vi "Write PinMap.vi"(8 "error in (no error)":errorcluster, 10 "PinMap":path, 11 "BML_DigiPattern_Generator in":refnum<class "DigiPattern_Generator.lvclass">) -> (0 "error out":errorcluster, 3 "BML_DigiPattern_Generator out":refnum<class "DigiPattern_Generator.lvclass">)   [LabVIEW 2018, in "DigiPattern_Generator.lvclass"]
uses:
  DigiPattern_Generator.lvclass
  DigiPattern_Generator.lvclass/DigiPattern_Generator.ctl
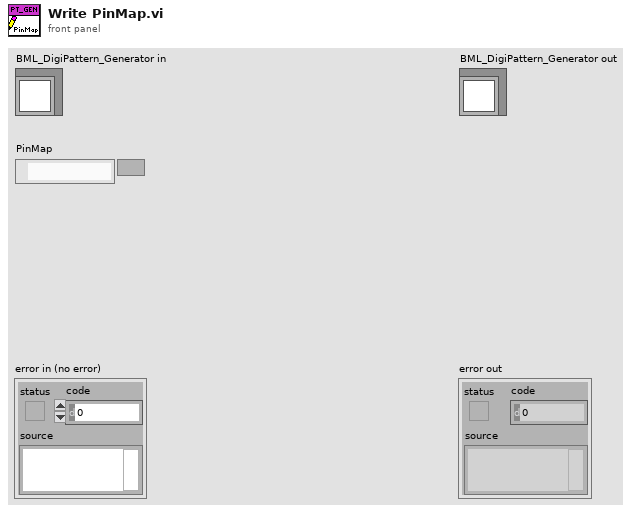
[diagram p1: front panel]
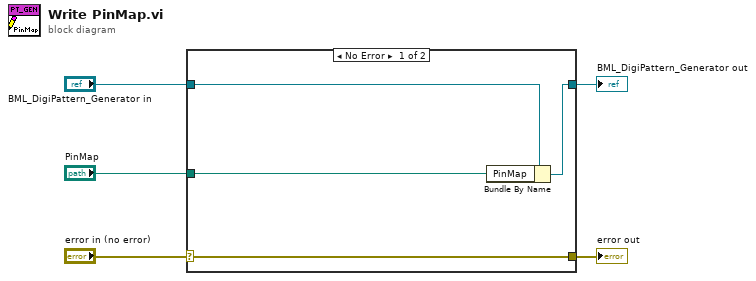
[diagram p0: block diagram]
diagram:
  n1 = case shown="No Error" "error in (no error)" {
    selector: "error in (no error)" -> [w9 w10]
    tunnel: [w9 w10] -> w4
    tunnel: [w7 w11] -> w2
    tunnel: "BML_DigiPattern_Generator in" -> [w8 w11]
    tunnel: "PinMap" -> [w6 _]
    frame No Error {
      n2 = Bundle By Name(cluster=w8, "PinMap"=w6) -> (w7:refnum<class "DigiPattern_Generator.lvclass">)
    }
    frame Error {
    }
  }
  "error out" <- w4
  "BML_DigiPattern_Generator out" <- w2
